vi "总磷质控流程.vi"(6 "队列输入TP":refnum<queue>, 9 "总磷":bool, 10 "总磷量程切换":enum32{"H", "L", "AUTO"}(ring)=enum."AUTO") -> (2 "总磷中断报警":bool, 3 "布尔":bool)   [LabVIEW 2016]
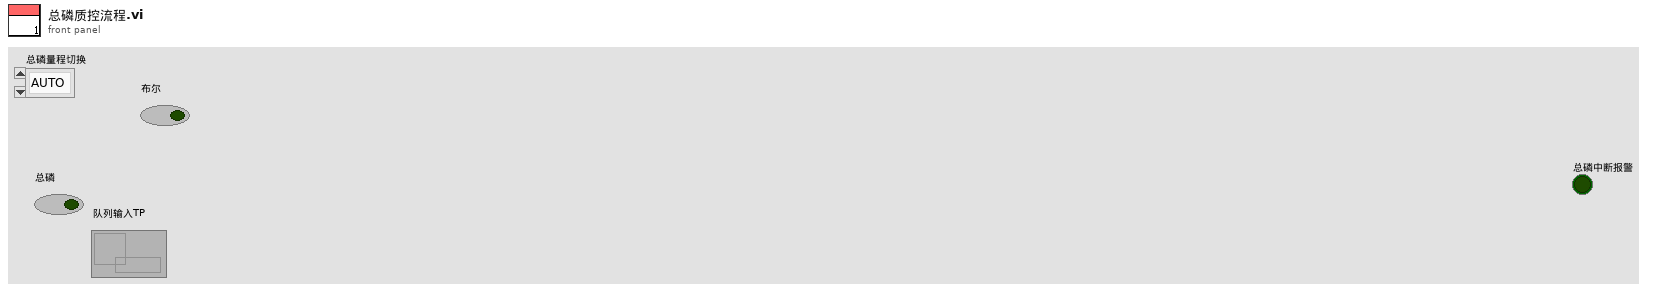
[diagram p1: front panel]
types:
  T1 = enum16{"待机", "启动氨氮水样", "氨氮测量中", "启动氨氮加标", "启动氨氮加标回收", "氨氮加标回收测量中", "启动总氮水样", "总氮测量中", "启动总氮加标", "启动总氮加标回收", "总氮加标回收测量中", "启动总磷水样", "总磷水样测量中", "启动总磷加标", "启动总磷加标回收", "总磷加标回收测量中", "结束"}
  T2 = cluster{"站号":u16, "量程切换":enum32{"H", "L", "AUTO"}, "控制命令":enum16{"启动测量", "标样核查", "零点核查", "跨度核查", "空白测试", "平行样测试", "加标回收", "空白校准", "标样校准", "初始化（清洗）", "停止测试", "仪器重启", "校时", "模式设置", "测量间隔设置"}, "模式设置":enum16{"待机", "连续模式", "周期模式", "定点模式", "受控模式", "手动模式"}, "测量间隔":u16}
  T3 = cluster{"时间标识":timestamp, "设备":string, "日志信息":string}
  T4 = cluster{"系统时间":timestamp, "工作状态":enum16{"空闲", "水样测试", "标样核查", "零点核查", "跨度核查", "空白测试", "平行样测试", "加标回收", "空白校准", "标样校准", "初始化（清洗）"}, "测量模式":enum16{"待机", "连续模式", "周期模式", "定点模式", "受控模式", "手动模式"}, "告警代码":enum16{"无告警", "缺试剂告警", "缺水样告警", "缺蒸馏水告警", "缺标液告警", "仪表漏液告警", "标定异常告警", "超量程告警", "加热异常", "低试剂预警", "超上限告警", "超下限告警", "仪表内部其他异常", "滴定异常告警", "电极异常告警", "量程切换告警", "参数设置告警", "PH电极电位异常", "电导率电极异常", "浊度光度异常", "溶解氧电极异常", "溶解氧光强异常", "温度异常告警", "PH异常告警", "溶解氧异常告警", "电导率异常告警", "浊度异常告警", "叶绿素异常告警", "藻密度异常告警", "蓝绿藻异常告警", "ORP异常告警", "氨氮异常告警", "清洁刷异常告警", "SD卡异常告警", "蓝牙异常告警", "Wifi异常告警", "流程异常告警"}, "故障代码":enum16{"无故障", "电机故障", "温度故障", "通讯故障", "滴定故障"}, "日志代码":u16, "软件版本":u16, "F0":sgl, "F1":sgl, "F2":sgl, "F3":sgl, "T":sgl, "H":sgl, "id":u16, "flowid":u16, "量程":u16, "总磷控温温度1":sgl, "营养盐控温温度2":sgl, "ADC":sgl}
  T5 = enum16{"空闲", "水样测试", "标样核查", "零点核查", "跨度核查", "空白测试", "平行样测试", "加标回收", "空白校准", "标样校准", "初始化（清洗）"}
  T6 = cluster{"因子编码":u32, "单位":u16, "标样参考值":sgl, "水样数据时间":timestamp, "水样实测值":sgl, "水样数据标识":string, "标样数据时间":timestamp, "标样实测值":sgl, "标样数据标识":string, "空白数据时间":timestamp, "空白实测值":sgl, "空白数据标识":string, "零点核查数据时间":timestamp, "零点核查实测值":sgl, "零点核查数据标识":string, "跨度核查数据时间":timestamp, "跨度核查实测值":sgl, "跨度核查数据标识":string, "加标回收数据时间":timestamp, "加标回收实测值":sgl, "加标回收数据标识":string, "平行样数据时间":timestamp, "平行样实测值":sgl, "平行样数据标识":string}
  T7 = cluster{"量程":dbl, "检出限":dbl, "加标前水样浓度":dbl, "加标后水样浓度":dbl, "加标水杯定容体积":dbl, "加标母液浓度":dbl, "加标体积":dbl, "加标回收率":dbl}
  T8 = cluster{"氨氮":u8, "总磷":u8, "总氮":u8, "CODMn":u8, "CODCr":u8}
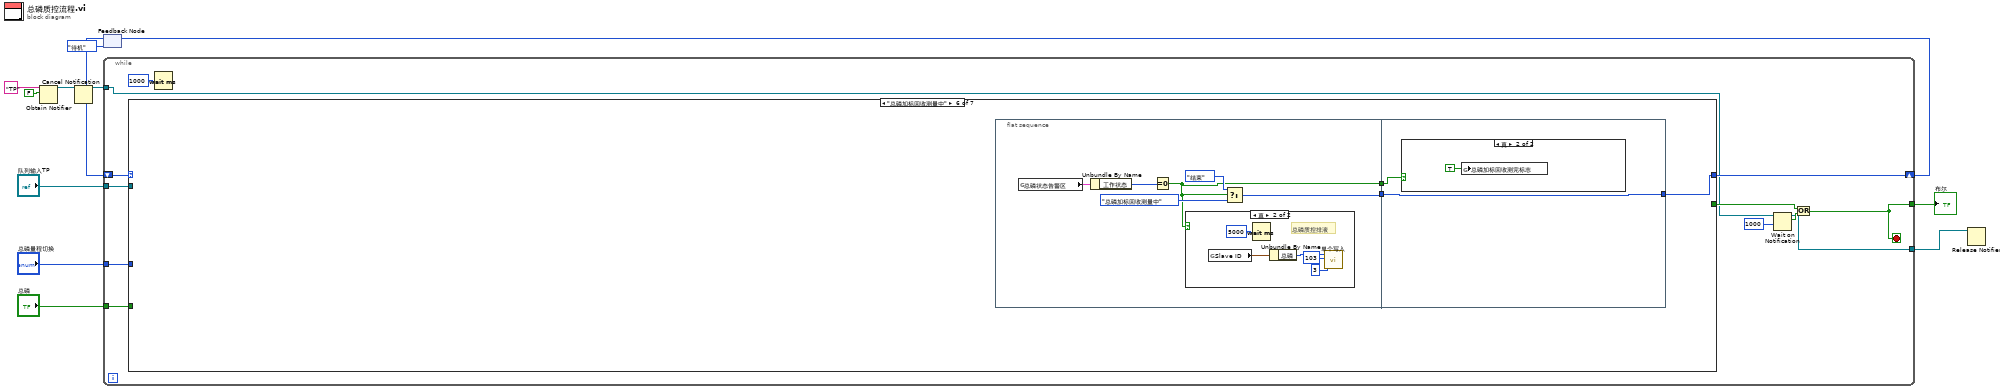
[diagram p0: block diagram]
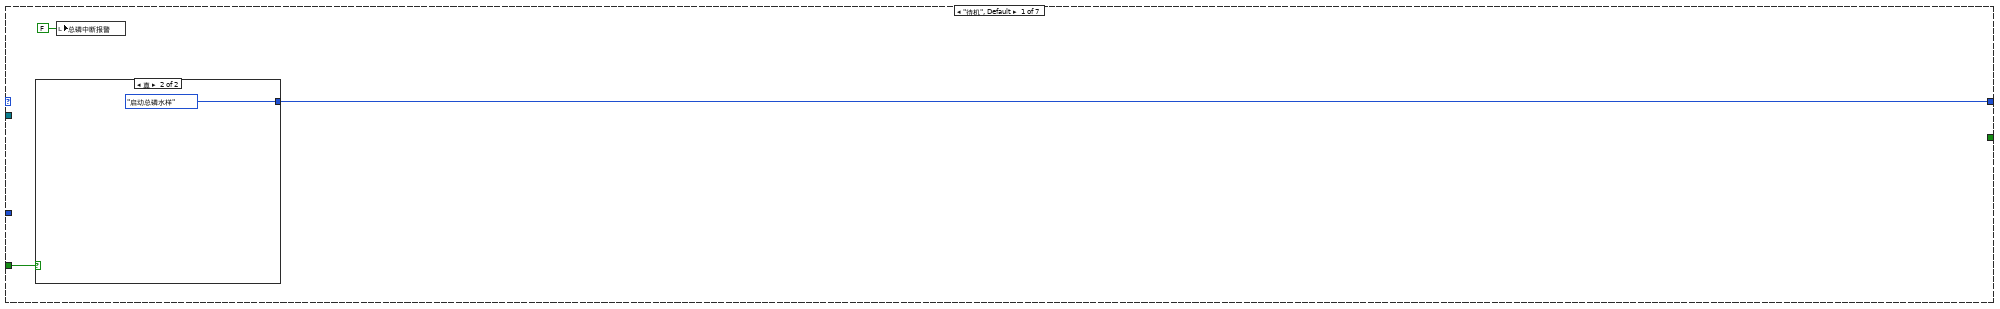
[diagram p2: hidden frame]
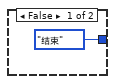
[diagram p3: hidden frame]
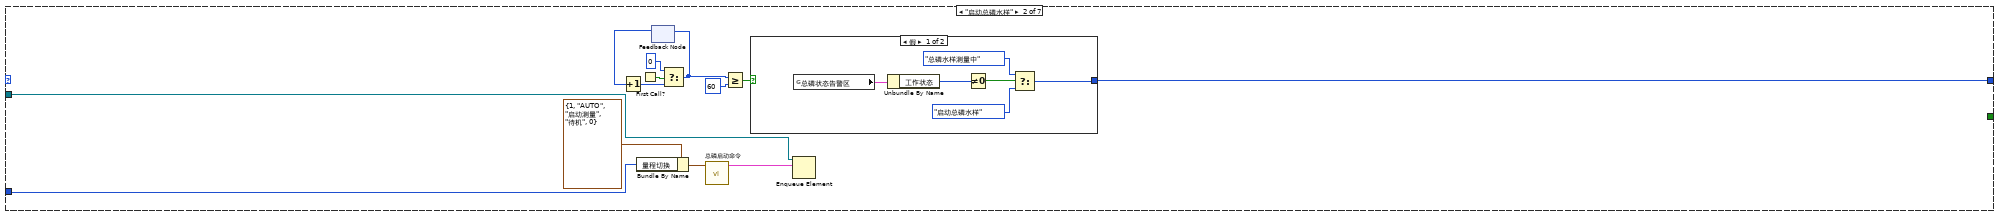
[diagram p4: hidden frame]
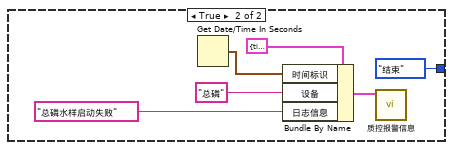
[diagram p5: hidden frame]
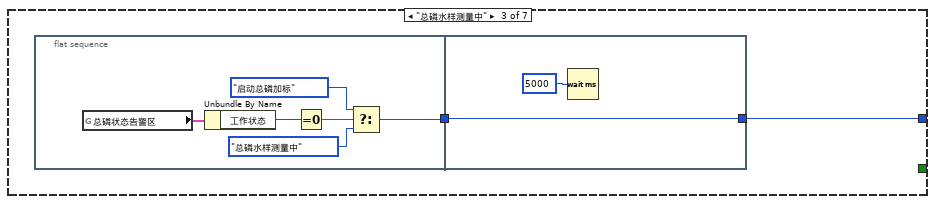
[diagram p6: hidden frame]
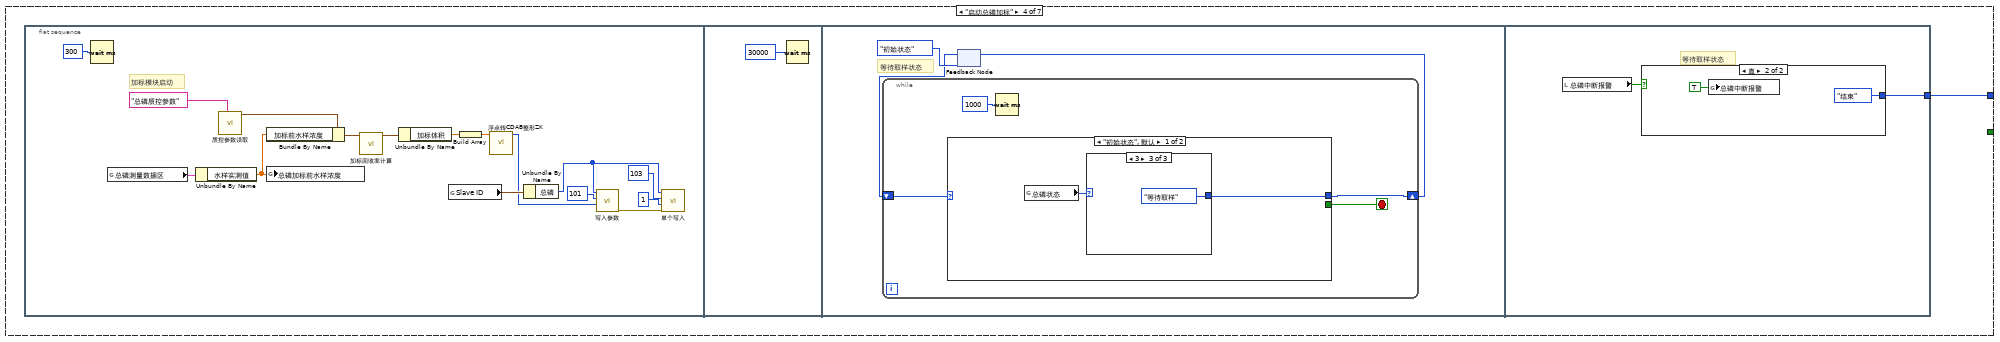
[diagram p7: hidden frame]
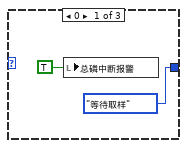
[diagram p8: hidden frame]
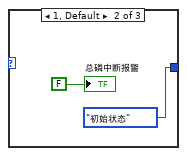
[diagram p9: hidden frame]
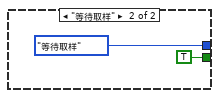
[diagram p10: hidden frame]
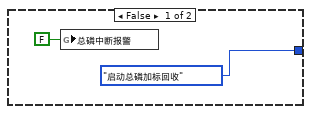
[diagram p11: hidden frame]
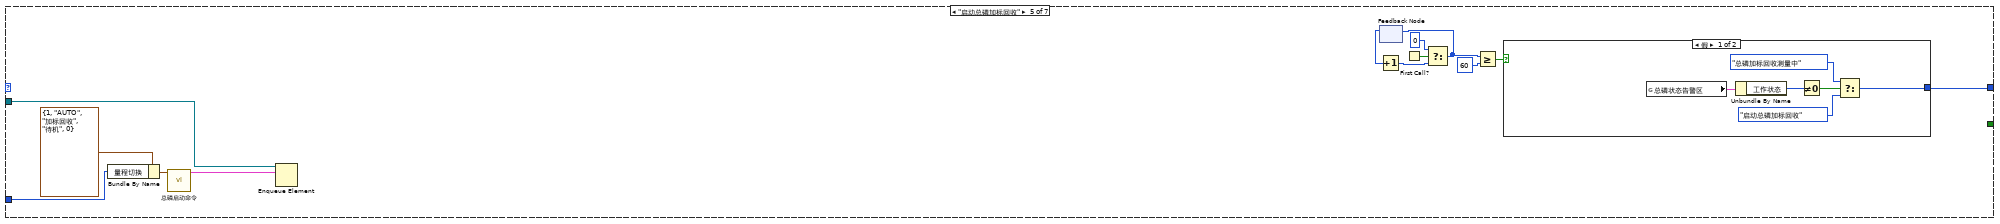
[diagram p12: hidden frame]
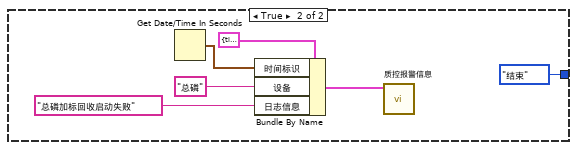
[diagram p13: hidden frame]
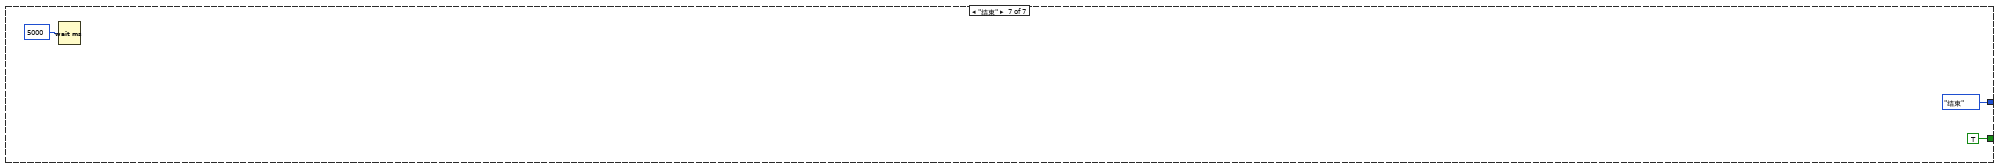
[diagram p16: hidden frame]
diagram:
  n1 = Obtain Notifier(name (unnamed)="TP" ("名称（未命名）"), notification data type=FALSE) -> (notifier out=w3:refnum<notifier>)  [unwired: 2 in, 2 out]
  n2 = Cancel Notification(0:w3) -> (8:w2:refnum<notifier>)  [unwired: 1 in, 2 out]
  n3 = feedback #1(T1."待机") -> (w6:T1)
  n4 = while {
    tunnel: "队列输入TP" -> [w22]
    tunnel: "总磷量程切换" -> [w21]
    tunnel: "总磷" -> [w24]
    tunnel: [w17] -> w11
    shift-right: [w23] -> w9
    shift-left: w6 -> [w19]
    tunnel: w2 -> [w15]
    tunnel: [w14] -> w1
    stop <- w17 stop-if-true
    n5 = case shown="\"总磷加标回收测量中\"" w19 {
      tunnel: [w27 w42 w55 w65 w110 w131 T1."结束"] -> w23
      tunnel: [_ _ _ _ _ _ TRUE] -> w16
      tunnel: w24 -> [w26 _ _ _ _ _ _]
      tunnel: w22 -> [_ w41 _ _ w109 _ _]
      tunnel: w21 -> [_ w40 _ _ w105 _ _]
      frame "待机", Default {
        n6 = case shown="真" w26 {
          tunnel: [T1."结束" T1."启动总磷水样"] -> w27
          frame False {
          }
          frame True {
          }
        }
        n7 = local write "总磷中断报警"(FALSE ("氨氮中断报警")) -> ()
      }
      frame "启动总磷水样" {
        n8 = Bundle By Name(cluster=T2 {"站号"=1, "量程切换"=enum."AUTO", "控制命令"=enum."启动测量", "模式设置"=enum."待机", "测量间隔"=0} ("参数"), "量程切换"=w40) -> (w32:T2)
        n9 = First Call?() -> (First Call?: T/F=w38:bool)
        n10 = feedback #2() -> (w37:i32)  [unwired: 1 in]
        n11 = Increment(x=w37) -> (x+1=w33:i32)
        n12 = Select(t=0, s=w38, f=w33) -> (s? t:f=w36:i32)
        n13 = feedback-in #2(w36) -> ()
        n14 = call "总磷启动命令.vi"("参数"=w32) -> ("启动命令"=w30:cluster{"命令":string, "data":variant})  [unwired: 10 in]
        n15 = Greater Or Equal?(x=w36, y=60) -> (x >= y?=w34:bool)
        n16 = case shown="假" w34 {
          tunnel: [w46 T1."结束"] -> w42
          frame False {
            n17 = global read "与总磷交互全局.vi" "总磷状态告警区"() -> (w43:T4)
            n18 = Unbundle By Name(w43) -> ("工作状态"=w48:T5)
            n19 = Not Equal To 0?(x=w48) -> (x != 0?=w47:bool)
            n20 = Select(t=T1."总磷水样测量中", s=w47, f=T1."启动总磷水样") -> (s? t:f=w46:T1)
          }
          frame True {
            n21 = Get Date/Time In Seconds() -> (seconds since 1Jan1904=w54:timestamp)
            n22 = Bundle By Name(cluster=T3 {"时间标识"=timestamp(0 s since 1904-01-01), "设备"="", "日志信息"=""} ("data in"), "时间标识"=w54, "设备"="总磷", "日志信息"="总磷水样启动失败") -> (w49:T3)
            n23 = call "质控报警信息.vi"("data in"=w49) -> ()  [unwired: 11 in]
          }
        }
        n24 = Enqueue Element(queue=w41, element=w30) -> ()  [unwired: 2 in, 3 out]
      }
      frame "总磷水样测量中" {
        n25 = flat-sequence {
          tunnel: [w57] -> w56
          tunnel: [w63] -> w55
          tunnel: w56 -> [w63]
          frame #0 {
            n26 = global read "与总磷交互全局.vi" "总磷状态告警区"() -> (w62:T4)
            n27 = Unbundle By Name(w62) -> ("工作状态"=w61:T5)
            n28 = Equal To 0?(x=w61) -> (x = 0?=w60:bool)
            n29 = Select(t=T1."启动总磷加标", s=w60, f=T1."总磷水样测量中") -> (s? t:f=w57:T1)
          }
          frame #1 {
            n30 = Wait (ms)(milliseconds to wait=u32 5000 ("等待时间（毫秒）")) -> ()  [unwired: 1 out]
          }
        }
      }
      frame "启动总磷加标" {
        n31 = flat-sequence {
          tunnel: [w100] -> w65
          frame #0 {
            # "加标模块启动"
            n32 = Wait (ms)(milliseconds to wait=u32 300 ("等待时间（毫秒）")) -> ()  [unwired: 1 out]
            n33 = global read "与总磷交互全局.vi" "总磷测量数据区"() -> (w74:T6)
            n34 = Unbundle By Name(w74) -> ("水样实测值"=w76:sgl)
            n35 = call "质控参数读取.vi"("section"="总磷质控参数") -> ("参数"=w79:T7)  [unwired: 9 in, 1 out]
            n36 = Bundle By Name(cluster=w79, "加标前水样浓度"=w76) -> (w80:T7)
            n37 = global write "水样浓度全局.vi" "总磷加标前水样浓度"(w76) -> ()
            n38 = call "加标回收率计算.vi"("参数"=w80) -> ("参数 out"=w78:T7)  [unwired: 9 in, 1 out]
            n39 = Unbundle By Name(w78) -> ("加标体积"=w77:dbl)
            n40 = global read "断电保存全局.vi" "Slave ID"() -> (w72:T8)
            n41 = Build Array(w77) -> (w73:dbl[])
            n42 = call "浮点转CDAB整形ZK.vi"("浮点数"=w73) -> ("CDAB整形输出"=w67:u16[])  [unwired: 10 in]
            n43 = Unbundle By Name(w72) -> ("总磷"=w66:u8)
            n44 = call "写入参数.vi"("values"=w67, "starting address"=u16 101, "Slave ID"=w66) -> ("error out"=w71:errorcluster)  [unwired: 8 in]
            n45 = call "单个写入.vi"("Error in"=w71, "value"=u16 1, "address"=u16 103, "Slave ID"=w66) -> ()  [unwired: 7 in, 1 out]
          }
          frame #1 {
            n46 = Wait (ms)(milliseconds to wait=u32 30000 ("等待时间（毫秒）")) -> ()  [unwired: 1 out]
          }
          frame #2 {
            # "等待取样状态"
            n47 = feedback #3(enum16{"初始状态", "等待取样"}."初始状态") -> (w84:enum16{"初始状态", "等待取样"})
            n48 = while {
              shift-right: [w88] -> w83
              shift-left: w84 -> [w89]
              stop <- w87 stop-if-true
              n49 = case shown="\"初始状态\", 默认" w89 {
                tunnel: [w91 enum16{"初始状态", "等待取样"}."等待取样"] -> w88
                tunnel: [_ TRUE] -> w87
                frame "初始状态", Default {
                  n50 = global read "加标回收状态全局变量.vi" "总磷状态"() -> (w90:u16)
                  n51 = case shown="3" w90 {
                    tunnel: [enum16{"初始状态", "等待取样"}."等待取样" enum16{"初始状态", "等待取样"}."初始状态" enum16{"初始状态", "等待取样"}."等待取样"] -> w91
                    frame 0 {
                      n52 = local write "总磷中断报警"(TRUE ("氨氮中断报警")) -> ()
                    }
                    frame 1, Default {
                      "总磷中断报警" <- FALSE ("总氮中断报警")
                    }
                    frame 3 {
                    }
                  }
                }
                frame "等待取样" {
                }
              }
              n53 = Wait (ms)(milliseconds to wait=u32 1000 ("等待时间（毫秒）")) -> ()  [unwired: 1 out]
            }
            n54 = feedback-in #3(w83) -> ()
          }
          frame #3 {
            # "等待取样状态"
            n55 = local read "总磷中断报警"() -> (w99:bool)
            n56 = case shown="真" w99 {
              tunnel: [T1."启动总磷加标回收" T1."结束"] -> w100
              frame False {
                n57 = global write "质控中断报警全局.vi" "总磷中断报警"(FALSE ("总磷中断报警")) -> ()
              }
              frame True {
                n58 = global write "质控中断报警全局.vi" "总磷中断报警"(TRUE ("总磷中断报警")) -> ()
              }
            }
          }
        }
      }
      frame "启动总磷加标回收" {
        n59 = Bundle By Name(cluster=T2 {"站号"=1, "量程切换"=enum."AUTO", "控制命令"=enum."加标回收", "模式设置"=enum."待机", "测量间隔"=0} ("参数"), "量程切换"=w105) -> (w107:T2)
        n60 = call "总磷启动命令.vi"("参数"=w107) -> ("启动命令"=w106:cluster{"命令":string, "data":variant})  [unwired: 10 in]
        n61 = Enqueue Element(queue=w109, element=w106) -> ()  [unwired: 2 in, 3 out]
        n62 = feedback #4() -> (w115:i32)  [unwired: 1 in]
        n63 = Increment(x=w115) -> (x+1=w114:i32)
        n64 = First Call?() -> (First Call?: T/F=w116:bool)
        n65 = Select(t=0, s=w116, f=w114) -> (s? t:f=w113:i32)
        n66 = feedback-in #4(w113) -> ()
        n67 = Greater Or Equal?(x=w113, y=60) -> (x >= y?=w111:bool)
        n68 = case shown="假" w111 {
          tunnel: [w121 T1."结束"] -> w110
          frame False {
            n69 = global read "与总磷交互全局.vi" "总磷状态告警区"() -> (w118:T4)
            n70 = Unbundle By Name(w118) -> ("工作状态"=w123:T5)
            n71 = Not Equal To 0?(x=w123) -> (x != 0?=w122:bool)
            n72 = Select(t=T1."总磷加标回收测量中", s=w122, f=T1."启动总磷加标回收") -> (s? t:f=w121:T1)
          }
          frame True {
            n73 = Get Date/Time In Seconds() -> (seconds since 1Jan1904=w129:timestamp)
            n74 = Bundle By Name(cluster=T3 {"时间标识"=timestamp(0 s since 1904-01-01), "设备"="", "日志信息"=""} ("data in"), "时间标识"=w129, "设备"="总磷", "日志信息"="总磷加标回收启动失败") -> (w124:T3)
            n75 = call "质控报警信息.vi"("data in"=w124) -> ()  [unwired: 11 in]
          }
        }
      }
      frame "总磷加标回收测量中" {
        n76 = flat-sequence {
          tunnel: [w137] -> w132
          tunnel: [w133] -> w130
          tunnel: [w145] -> w131
          tunnel: w132 -> [w145]
          tunnel: w130 -> [w144]
          frame #0 {
            n77 = global read "与总磷交互全局.vi" "总磷状态告警区"() -> (w134:T4)
            n78 = Unbundle By Name(w134) -> ("工作状态"=w138:T5)
            n79 = Equal To 0?(x=w138) -> (x = 0?=w133:bool)
            n80 = case shown="真" w133 {
              frame False {
              }
              frame True {
                # "总磷质控排液"
                n81 = global read "断电保存全局.vi" "Slave ID"() -> (w142:T8)
                n82 = Wait (ms)(milliseconds to wait=u32 5000 ("等待时间（毫秒）")) -> ()  [unwired: 1 out]
                n83 = Unbundle By Name(w142) -> ("总磷"=w141:u8)
                n84 = call "单个写入.vi"("value"=u16 3, "address"=u16 103, "Slave ID"=w141) -> ()  [unwired: 8 in, 1 out]
              }
            }
            n85 = Select(t=T1."结束", s=w133, f=T1."总磷加标回收测量中") -> (s? t:f=w137:T1)
          }
          frame #1 {
            n86 = case shown="真" w144 {
              frame False {
              }
              frame True {
                n87 = global write "质控测完标志全局 1.vi" "总磷加标回收测完标志"(TRUE) -> ()
              }
            }
          }
        }
      }
      frame "结束" {
        n88 = Wait (ms)(milliseconds to wait=u32 5000 ("等待时间（毫秒）")) -> ()  [unwired: 1 out]
      }
    }
    n89 = Wait (ms)(milliseconds to wait=u32 1000 ("等待时间（毫秒）")) -> ()  [unwired: 1 out]
    n90 = Wait on Notification(notifier=w15, timeout in ms (-1)=1000 ("超时毫秒(-1)")) -> (notifier out=w14:refnum<notifier>, notification=w18:bool)  [unwired: 2 in, 2 out]
    n91 = Or(x=w16, y=w18) -> (x .or. y?=w17:bool)
  }
  "布尔" <- w11
  n92 = feedback-in #1(w9) -> ()
  n93 = Release Notifier(notifier=w1) -> ()  [unwired: 2 in, 3 out]
